vi "Run.vi"(8 "error in (no error)":errorcluster, 9 "s on last turn":dbl=0.3439976484514773, 10 "Maze (0: Empty, -1: Enemy. >0: Teammate":i32[][](array[numeric])=[[16, 0, 18], [0, 14, 0], [0, 0, 0]], 11 "Mother In":refnum<class "Formics.lvclass">=refnum) -> (0 "error out":errorcluster, 1 "Direction":T1=enum."SE", 2 "Action":T2=enum."Replicate", 3 "Mother Out":refnum<class "Formics.lvclass">, 4 "Replicated":refnum<class "Square.lvclass">)   [LabVIEW 2014, in "Formics.lvclass"]
uses:
  Formics.lvclass
  SquareBattle Arena/Action Enum.ctl
  SquareBattle Arena/Direction Enum.ctl
  Square.lvclass
  Protector/Protector.lvclass
  Formics.lvclass/Formics.ctl
  Attack Options.ctl
  SquareBattle Arena/SquareBattle Arena.lvclass
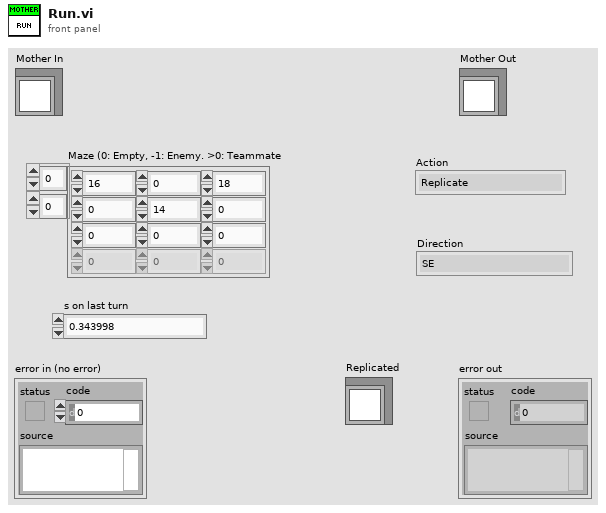
[diagram p1: front panel]
types:
  T1 = typedef "SquareBattle Arena.lvlib/SquareBattle Arena.lvclass/Direction Enum.ctl" = enum16{"NW", "N", "NE", "E", "SE", "S", "SW", "W"}
  T2 = typedef "SquareBattle Arena.lvlib/SquareBattle Arena.lvclass/Action Enum.ctl" = enum16{"Wait", "Move", "Attack", "Replicate"}
  T3 = enum16{"Queen", "Daughter", "Kamikazee", "Coward", "Migrate", "Line Up"}
  T4 = typedef "Formics.lvclass/Attack Options.ctl" = enum16{"Attack", "Run", "Distract"}
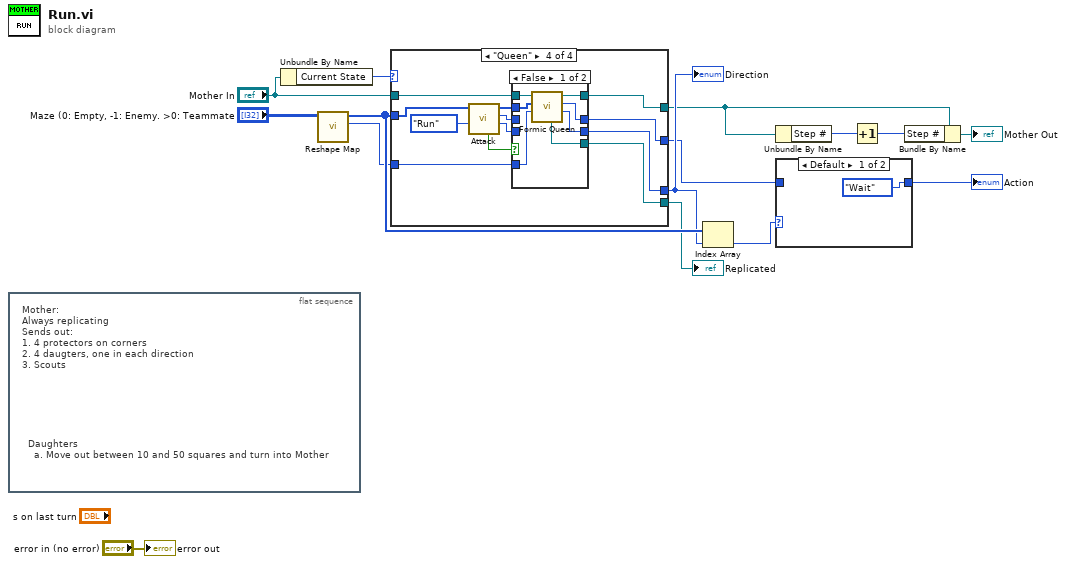
[diagram p0: block diagram]
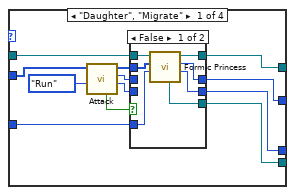
[diagram p2: hidden frame]
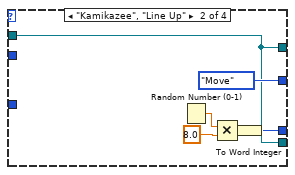
[diagram p4: hidden frame]
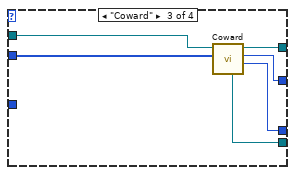
[diagram p5: hidden frame]
diagram:
  n1 = flat-sequence {
    frame #0 {
      # "Daughters\n  a. Move out between 10 and 50 squares and turn into Mother"
      # "Mother:\nAlways replicating\nSends out:\n1. 4 protectors on corners\n2. 4 daugters, one in each direction\n3. Scouts"
    }
  }
  n2 = Unbundle By Name("Mother In") -> ("Current State"=w9:T3)
  n3 = call "Reshape Map.vi"("Maze (0: Empty, -1: Enemy. >0: Teammate"="Maze (0: Empty, -1: Enemy. >0: Teammate") -> ("SelfID"=w10:i32, "Map"=w11:i32[])  [unwired: 9 in]
  n4 = case shown="\"Queen\"" w9 {
    tunnel: "Mother In" -> [w27 w40 w49 w61]
    tunnel: [w26 w40 w48 w60] -> w6
    tunnel: w11 -> [w25 _ w44 w58]
    tunnel: w10 -> [w20 _ _ w56]
    tunnel: [w16 w38 w46 w51] -> w7
    tunnel: [w22 w40 w45 w54] -> w5
    tunnel: [w21 Action_Enum."Move" ("Action") w47 w55] -> w4
    frame "Daughter", "Migrate" {
      n5 = call "Attack.vi"("Attack?"=Attack_Options."Run", "Maze (0: Empty, -1: Enemy. >0: Teammate"=w25) -> ("Direction"=w17:i32, "Action"=w18:T2, "Maze (0: Empty, -1: Enemy. >0: Teammate 2"=w24:i32[], "Enemy Found?"=w19:bool)  [unwired: 4 in, 2 out]
      n6 = case shown="False" w19 {
        tunnel: w27 -> [w34 w37]
        tunnel: [w33 w37] -> w26
        tunnel: w24 -> [w32 _]
        tunnel: [w31 w37] -> w22
        tunnel: [w30 w36] -> w21
        tunnel: w20 -> [w29 _]
        tunnel: w18 -> [_ w36]
        tunnel: w17 -> [_ w35]
        tunnel: [w28 w35] -> w16
        frame False {
          n7 = call "Formic Princess.vi"("SelfID"=w29, "Map"=w32, "Mother in"=w34) -> ("Direction"=w28:T1, "Action"=w30:T2, "Mother out"=w33:refnum<class "Formics.lvclass">, "Replicated Class"=w31:refnum<class "Formics.lvclass">)  [unwired: 4 in, 1 out]
        }
        frame True {
        }
      }
    }
    frame "Kamikazee", "Line Up" {
      n8 = Random Number (0-1)() -> (number: 0 to 1=w42:dbl)
      n9 = Multiply(x=w42, y=8.0) -> (x*y=w39:dbl)
      n10 = To Word Integer(number=w39) -> (16bit integer=w38:i16)
    }
    frame "Coward" {
      n11 = call-dynamic "Coward.vi"("Map"=w44, "Mother In"=w49) -> ("Direction"=w46:T1, "Action"=w47:T2, "Mother Out"=w48:refnum<class "Formics.lvclass">, "Replicated"=w45:refnum<class "Square.lvclass">)  [unwired: 5 in, 1 out]
    }
    frame "Queen" {
      n12 = call "Attack.vi"("Attack?"=Attack_Options."Run", "Maze (0: Empty, -1: Enemy. >0: Teammate"=w58) -> ("Direction"=w52:i32, "Action"=w53:T2, "Maze (0: Empty, -1: Enemy. >0: Teammate 2"=w57:i32[], "Enemy Found?"=w50:bool)  [unwired: 4 in, 2 out]
      n13 = case shown="False" w50 {
        tunnel: w61 -> [w68 w69]
        tunnel: [w67 w69] -> w60
        tunnel: w57 -> [w66 _]
        tunnel: w56 -> [w65 _]
        tunnel: [w64 w71] -> w55
        tunnel: [w63 w69] -> w54
        tunnel: w53 -> [_ w71]
        tunnel: w52 -> [_ w70]
        tunnel: [w62 w70] -> w51
        frame False {
          n14 = call "Formic Queen.vi"("SelfID"=w65, "Map"=w66, "Mother in"=w68) -> ("Direction"=w62:T1, "Action"=w64:T2, "Mother out"=w67:refnum<class "Formics.lvclass">, "Replicated Class"=w63:refnum<class "Formics.lvclass">)  [unwired: 4 in, 1 out]
        }
        frame True {
        }
      }
    }
  }
  "Direction" <- w7
  "Replicated" <- w5
  n15 = Index Array(array=w11, index=w7) -> (element=w14:i32)
  n16 = Unbundle By Name(w6) -> ("Step #"=w2:i32)
  n17 = case shown="Default" w14 {
    tunnel: w4 -> [_ w73]
    tunnel: [Action_Enum."Wait" ("Action") w73] -> w13
    frame Default {
    }
    frame -1, 0 {
    }
  }
  "Action" <- w13
  n18 = Increment(x=w2) -> (x+1=w1:i32)
  n19 = Bundle By Name(cluster=w6, "Step #"=w1) -> (→"Mother Out":refnum<class "Formics.lvclass">)
  "error out" <- "error in (no error)"
